vi "Compute.vi"(8 "error in (no error)":errorcluster, 9 "Data Channels":T1, 10 "x-var":dbl, 11 "Polarization in":refnum<class "Polarization.lvclass">) -> (0 "error out":errorcluster, 1 "Add'l Data Channels":T1, 3 "Polarization out":refnum<class "Polarization.lvclass">)   [LabVIEW 2009, in "Polarization.lvclass"]
doc: "Given a data channel and an x-coordinate, compute and return one or more new data channels."
uses:
  Polarization.lvclass
  Instruments/Utility Classes/Readable/Data Channels.ctl
  Instruments/Utility Classes/Readable/Data Channel.ctl
  Instruments/Utility Classes/Readable/Data Point.ctl
  Instruments/Utility Classes/Readable/Readable.lvclass
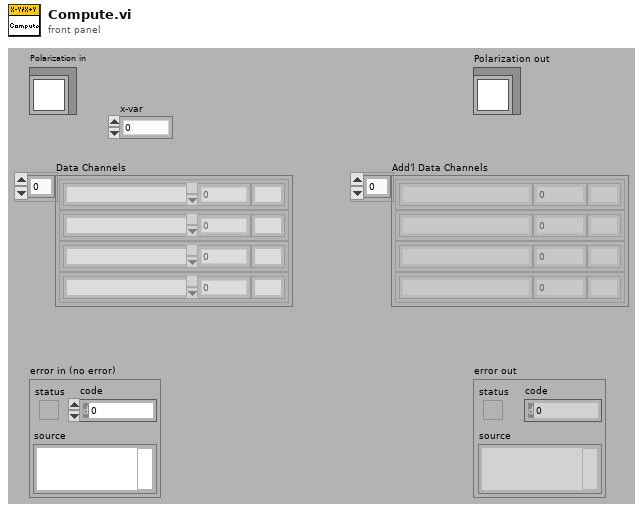
[diagram p1: front panel]
types:
  T1 = typedef "Readable.lvclass/Data Channels.ctl" = T2[]
  T2 = typedef "Readable.lvclass/Data Channel.ctl" = cluster{"Name":string, "Data Point":T3, "Unit":string}
  T3 = typedef "Readable.lvclass/Data Point.ctl" = dbl
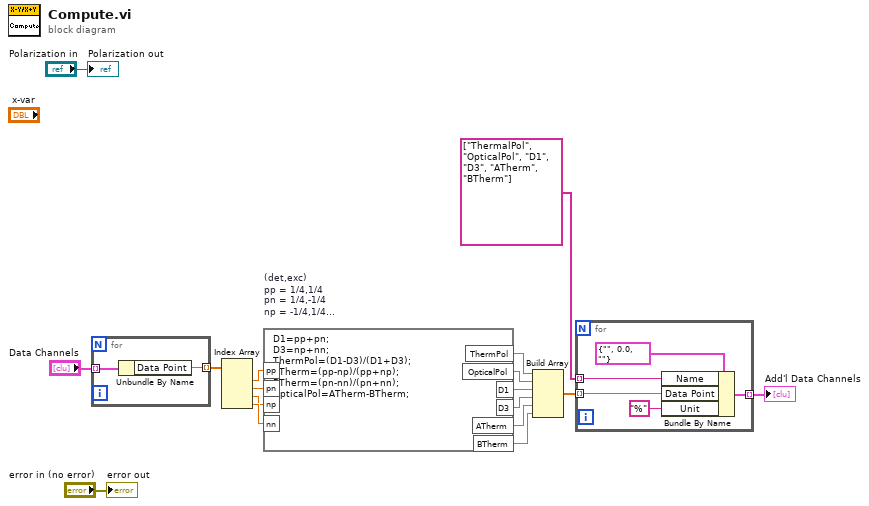
[diagram p0: block diagram]
diagram:
  n1 = for {
    tunnel: "Data Channels" -> [w19] mode=indexing
    tunnel: [w18] -> w14 mode=indexing
    n2 = Unbundle By Name(w19) -> ("Data Point"=w18:T3)
  }
  n3 = Index Array(array=w14) -> (element #1=w13:T3, element #2=w12:T3, element #3=w1:T3, element #4=w11:T3)  [unwired: 4 in]
  n4 = formula code="D1=pp+pn;\nD3=np+nn;\nThermPol=(D1-D3)/(D1+D3);\nATherm=(pp-np)/(pp+np);\nBTherm=(pn-nn)/(pn+nn);\nOpticalPol=ATherm-BTherm;" "(det,exc)\npp = 1/4,1/4\npn = 1/4,-1/4\nnp = -1/4,1/4\nnn = -1/4,-1/4"("pp"=w13, "pn"=w12, "np"=w1, "nn"=w11) -> ("D1"=w8:dbl, "D3"=w7:dbl, "ThermPol"=w10:dbl, "ATherm"=w6:dbl, "BTherm"=w5:dbl, "OpticalPol"=w9:dbl)
  n5 = Build Array(w10, w9, w8, w7, w6, w5) -> (w4:dbl[])
  n6 = for {
    tunnel: w4 -> [w23] mode=indexing
    tunnel: string[] ["ThermalPol", "OpticalPol", "D1", "D3", "ATherm", "BTherm"] -> [w22] mode=indexing
    tunnel: [w21] -> w2 mode=indexing
    n7 = Bundle By Name(cluster=T2 {"Name"="", "Data Point"=0.0, "Unit"=""} ("Data Channel"), "Name"=w22, "Data Point"=w23, "Unit"="%") -> (w21:T2)
  }
  "Add'l Data Channels" <- w2
  "error out" <- "error in (no error)"
  "Polarization out" <- "Polarization in"
